vi "Get File Extension (String).vi"(10 "File Path":string) -> (2 "File Name":string, 3 "File Extension":string)   [LabVIEW 2017]
doc: "Returns the file extension, without the period (.), of a file you specify in <b>File Path</b>."
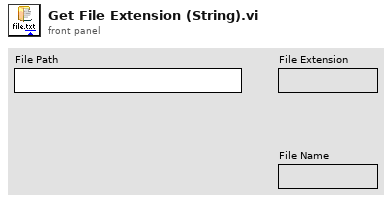
[diagram p1: front panel]
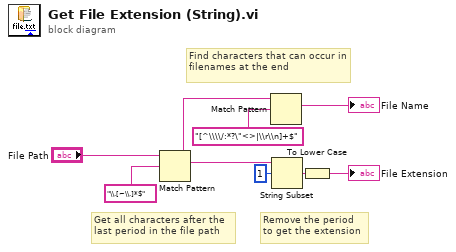
[diagram p0: block diagram]
diagram:
  # "Find characters that can occur in filenames at the end"
  # "Remove the period \nto get the extension"
  # "Get all characters after the \nlast period in the file path"
  n1 = Match Pattern(string="File Path", regular expression="\\.[~\\.]*$") -> (before substring=w4:string, match substring=w8:string)  [unwired: 3 out]
  n2 = Match Pattern(string=w4, regular expression="[^\\\\/:*?\"<>|\\r\\n]+$") -> (match substring=→"File Name":string)  [unwired: 4 out]
  n3 = String Subset(string=w8, offset (0)=1) -> (substring=w5:string)  [unwired: 1 out]
  n4 = To Lower Case(string=w5) -> (all lower case string=→"File Extension":string)
